vi "Create NI 9225.vi"(8 "error in":errorcluster, 11 "channel settings":T1[](array[typedef])) -> (0 "error out":errorcluster, 3 "NI 9225 out":refnum<class "NI 9225.lvclass">)   [LabVIEW 2017, in "Scan Engine Scripting.lvlib" / "NI 9225.lvclass"]
uses:
  NI 9225.lvclass
  Mode Classes/Controls/analog channel settings.ctl
  Mode Classes/Analog Input Vrms Mode/Analog Input Vrms Mode.lvclass
  C:/dev/github.com/debryant/niveristand-scan-engine-ethercat-custom-device/Custom Device Source/Scripting/Modules/Mode Classes/Mode/Mode.lvclass
  4ab162af-d640-44eb-9977-177cf6a3db57.vi
  Scan Engine Scripting.lvlib
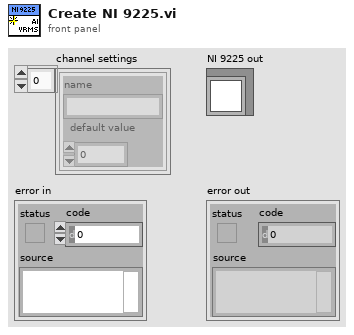
[diagram p1: front panel]
types:
  T1 = typedef "Scan Engine Scripting.lvlib/analog channel settings.ctl" = cluster{"name":string, "default value":dbl}
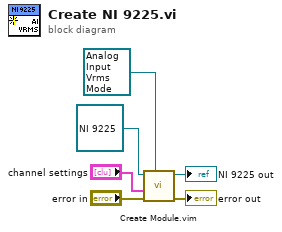
[diagram p0: block diagram]
diagram:
  n1 = call "Create Module.vim"("mode in"=refnum<class "Analog Input Vrms Mode.lvclass"> refnum ("Scan Engine Scripting.lvlib:Analog Input Vrms Mode.lvclass"), "error in"="error in", "channel settings"="channel settings", "module in"=refnum<class "NI 9225.lvclass"> refnum ("Scan Engine Scripting.lvlib:NI 9225.lvclass")) -> ("error out"=→"error out":errorcluster, "module out"=→"NI 9225 out":refnum<class "NI 9225.lvclass">)  [unwired: 6 in]
